vi "_Parse SEM Extreme Result.vi"(8 "error in (no error)":errorcluster, 10 "Input String":string, 11 "VISA resource name":refnum<visa-resource-name>) -> (0 "error out":errorcluster, 1 "Measurement Result":T1 {"TX Power Max" format="%^.3e"; "TX Power Min" format="%^.3e"; "OBW" format="%^.3e"; "Out Of Tolerance" format="%^.3e"}, 2 "Reliability":i32, 3 "VISA resource name out":refnum<visa-resource-name>)   [LabVIEW 2015, in "Rohde&Schwarz CMXP NR FR2 Measurement.lvlib"]
uses:
  <instrlib>/Rohde&Schwarz CMXP NR FR2 Measurement/Rohde&Schwarz CMXP NR FR2 Measurement.lvlib
  <instrlib>/Rohde&Schwarz CMXP NR FR2 Measurement/Private/rsidr_core.llb/rsidr_core.lvlib
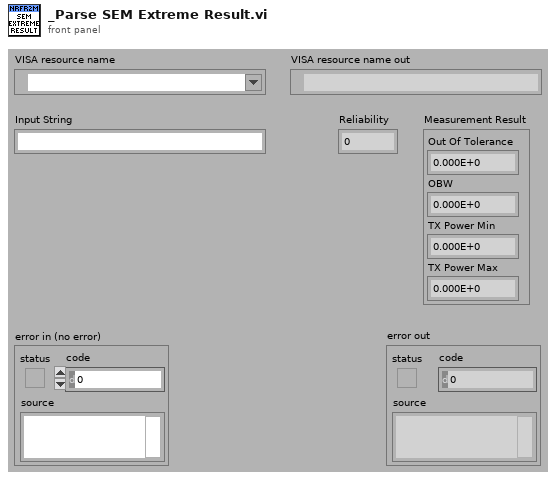
[diagram p1: front panel]
types:
  T1 = cluster{"Out Of Tolerance":dbl, "OBW":dbl, "TX Power Min":dbl, "TX Power Max":dbl}
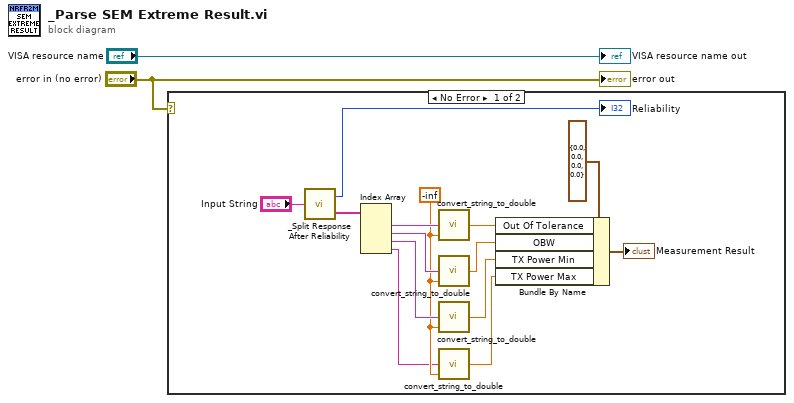
[diagram p0: block diagram]
diagram:
  n1 = case shown="No Error" "error in (no error)" {
    frame No Error {
      w6 = -inf
      n2 = call <instrlib>:"_Split Response After Reliability.vi"("Input String"="Input String") -> ("Response out"=w11:string[], "Reliability out"=→"Reliability":i32)
      n3 = Index Array(array=w11) -> (element #1=w10:string, element #2=w9:string, element #3=w8:string, element #4=w5:string)  [unwired: 4 in]
      n4 = call <instrlib>:"convert_string_to_double.vi"("default (0)"=w6, "String in"=w10) -> ("double value out"=w16:dbl)  [unwired: 3 in]
      n5 = call <instrlib>:"convert_string_to_double.vi"("default (0)"=w6, "String in"=w9) -> ("double value out"=w15:dbl)  [unwired: 3 in]
      n6 = call <instrlib>:"convert_string_to_double.vi"("default (0)"=w6, "String in"=w8) -> ("double value out"=w14:dbl)  [unwired: 3 in]
      n7 = call <instrlib>:"convert_string_to_double.vi"("default (0)"=w6, "String in"=w5) -> ("double value out"=w4:dbl)  [unwired: 3 in]
      n8 = Bundle By Name(cluster=T1 {"Out Of Tolerance"=0.0, "OBW"=0.0, "TX Power Min"=0.0, "TX Power Max"=0.0} ("Measurement Result"), "Out Of Tolerance"=w16, "OBW"=w15, "TX Power Min"=w14, "TX Power Max"=w4) -> (→"Measurement Result":T1)
    }
    frame Error {
    }
  }
  "error out" <- "error in (no error)"
  "VISA resource name out" <- "VISA resource name"
